vi "samp_s1_2018.vi"() -> ()   [LabVIEW 2017]
uses:
  <userlib>/Open_device_2017.llb/Select_Instr.ctl
panel:
  in  "Channel":u8
  out "Read counter":i32
  out "error out":errorcluster
  out "Opened":bool
  in  "stop":bool
  out "read buffer":string
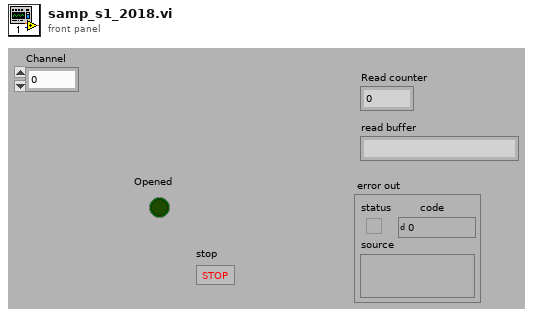
[diagram p1: front panel]
types:
  T1 = typedef "Select_Instr.ctl" = string
  T2 = cluster{"VISA resource name 1":refnum<visa-resource-name>, "VISA resource name 2":refnum<visa-resource-name>}
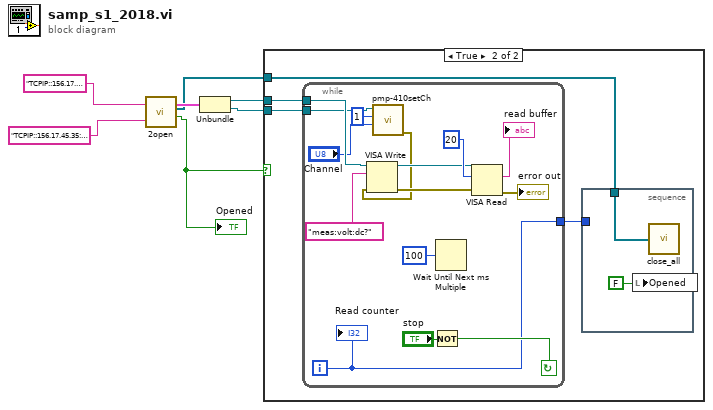
[diagram p0: block diagram]
diagram:
  n1 = call <userlib>:"2open.vi"("VISA resource name 1"=T1 "TCPIP::156.17.45.35::inst27::INSTR" ("Select_Instrument"), "VISA resource name 2"=T1 "TCPIP::156.17.45.35::inst104::INSTR" ("Select_Instrument")) -> ("InstrCluster"=w6:T2, "InstrArray"=w4:refnum<visa-resource-name>[], "Open OK (true)"=w5:bool)  [unwired: 1 out]
  "Opened" <- w5
  n2 = Unbundle(w6) -> ("VISA resource name 1"=w7:refnum<visa-resource-name>, "VISA resource name 2"=w1:refnum<visa-resource-name>)
  n3 = case shown="True" w5 {
    tunnel: w7 -> [_ w11]
    tunnel: w4 -> [_ w9]
    tunnel: w1 -> [_ w8]
    frame False {
    }
    frame True {
      n4 = while {
        tunnel: w11 -> [w28]
        tunnel: [w21] -> w10
        tunnel: w8 -> [w17]
        i -> [w21]
        stop <- w23 continue-if-true
        n5 = call <userlib>:"pmp-410setCh.vi"("Channel"="Channel", "Slave#"=u8 1, "VISA Refnum in"=w17) -> ("error out"=w16:errorcluster)  [unwired: 7 in, 1 out]
        n6 = VISA Write(VISA resource name=w28, write buffer="meas:volt:dc?" ("write buffer (\"\")"), error in (no error)=w16) -> (VISA resource name out=w19:refnum<visa-resource-name>, error out=w18:errorcluster)  [unwired: 1 out]
        n7 = Not(x="stop") -> (.not. x?=w23:bool)
        n8 = Wait Until Next ms Multiple(millisecond multiple=u32 100) -> ()  [unwired: 1 out]
        n9 = VISA Read(VISA resource name=w19, byte count=u32 20 ("byte count (0)"), error in (no error)=w18) -> (read buffer=→"read buffer":string, error out=→"error out":errorcluster)  [unwired: 2 out]
        "Read counter" <- w21
      }
      n10 = stacked-sequence {
        tunnel: w10 -> [_]
        tunnel: w9 -> [w12]
        frame #0 {
          n11 = local write "Opened"(FALSE) -> ()
          n12 = call <userlib>:"close_all.vi"("OpenRes"=w12) -> ()  [unwired: 1 out]
        }
      }
    }
  }
